vi "COMMUNICATE_WITH_DEVICE (SubVI).vi"(8 "error in (no error)":errorcluster, 10 "created command":string, 11 "VISA Refnum in":refnum<visa-resource-name>) -> (0 "error out":errorcluster, 3 "Measured Output Value":dbl)   [LabVIEW 2020]
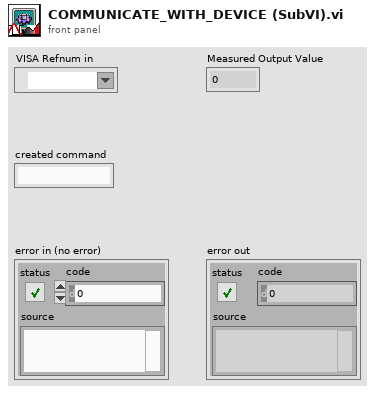
[diagram p1: front panel]
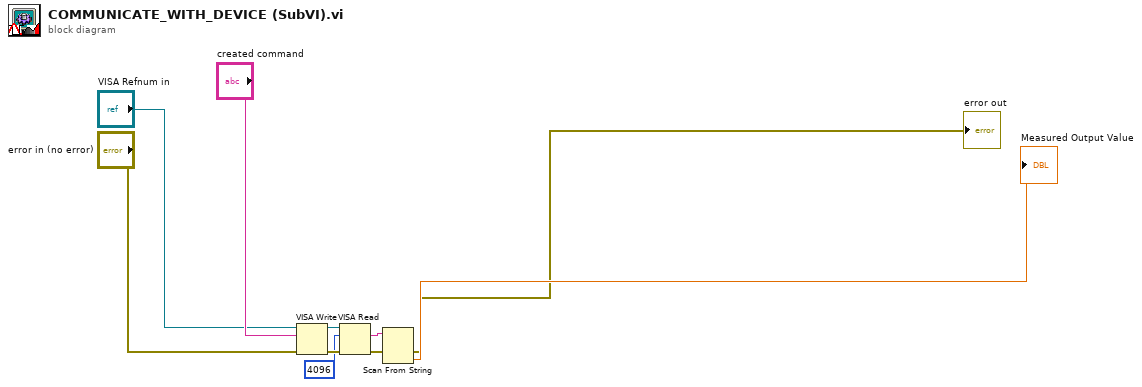
[diagram p0: block diagram]
diagram:
  n1 = VISA Write(VISA resource name="VISA Refnum in", write buffer="created command", error in (no error)="error in (no error)") -> (VISA resource name out=w3:refnum<visa-resource-name>, error out=w2:errorcluster)  [unwired: 1 out]
  n2 = VISA Read(VISA resource name=w3, byte count=u32 4096, error in (no error)=w2) -> (read buffer=w6:string, error out=w9:errorcluster)  [unwired: 2 out]
  n3 = Scan From String(input string=w6, error in=w9) -> (error out=→"error out":errorcluster, output 1=→"Measured Output Value":dbl)  [unwired: 3 in, 2 out]
